vi "Select_Table_Vaule.vi"(6 "Boolean":bool, 8 "Vaule":string, 9 "Action":string, 11 "Table":string[][](array[string])) -> (0 "Result":bool, 3 "vaule":string[](array[string]))   [LabVIEW 2017]
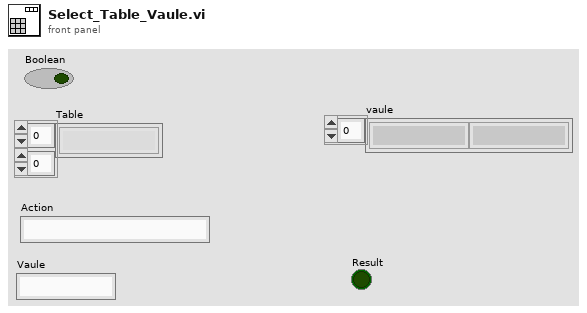
[diagram p1: front panel]
types:
  T1 = typedef "HD Config.ctl" = cluster{" PC":cluster{"PC Address":u8[], "PC Port":i32}, "FCO":cluster{"COM":refnum<visa-resource-name>, "Baudrate":u32}, "DC Power ":cluster{"COM":refnum<visa-resource-name>, "Baudrate":u32}, "PW3336":cluster{"COM":refnum<visa-resource-name>, "Baudrate":u32}, "Lefoo":cluster{"COM":refnum<visa-resource-name>, "Baudrate":u32}, "Tempt&Hum":cluster{"COM":refnum<visa-resource-name>, "Baudrate":u32}, "DIPC":cluster{"COM":refnum<visa-resource-name>}, "Daemon":cluster{"IP Address":string, "Port":u16, "Retry":u16}, "NFC_Cmd":cluster{"COM":refnum<visa-resource-name>, "Baudrate":u32}, "Fail_resume_mode":bool, "GRR":bool, "NFC _Serial":cluster{"COM":refnum<visa-resource-name>, "Baudrate":u32}}
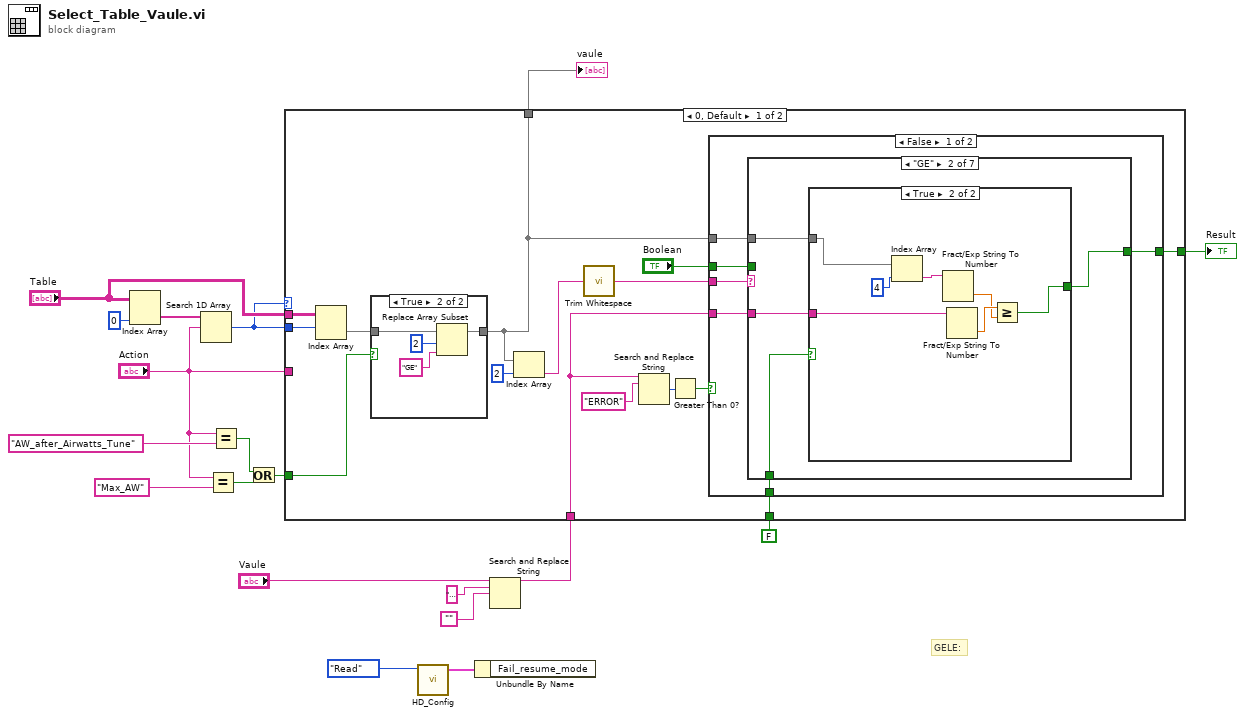
[diagram p0: block diagram]
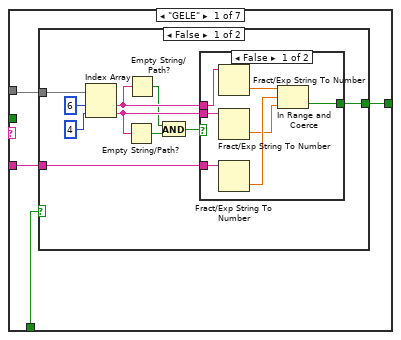
[diagram p3: hidden frame]
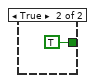
[diagram p4: hidden frame]
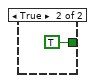
[diagram p5: hidden frame]
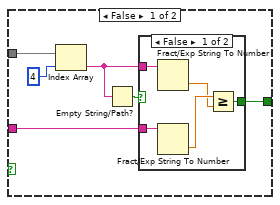
[diagram p6: hidden frame]
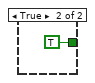
[diagram p7: hidden frame]
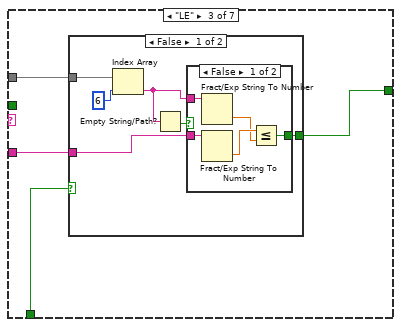
[diagram p8: hidden frame]
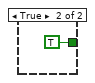
[diagram p9: hidden frame]
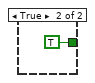
[diagram p10: hidden frame]
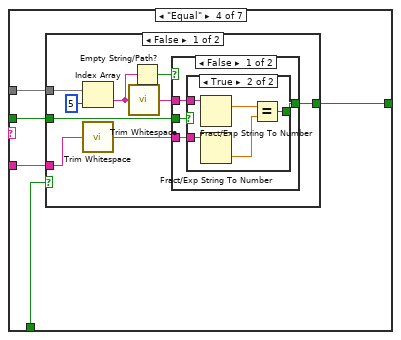
[diagram p11: hidden frame]
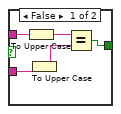
[diagram p12: hidden frame]
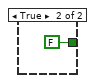
[diagram p13: hidden frame]
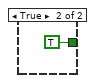
[diagram p14: hidden frame]
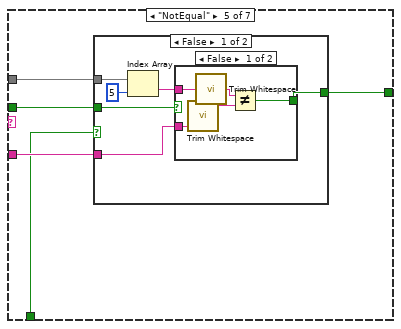
[diagram p15: hidden frame]
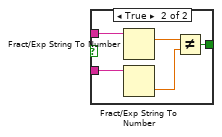
[diagram p16: hidden frame]
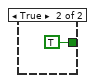
[diagram p17: hidden frame]
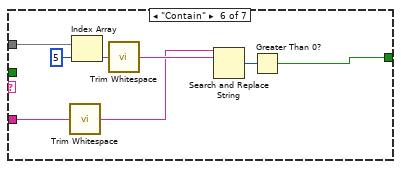
[diagram p18: hidden frame]
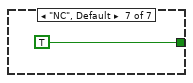
[diagram p19: hidden frame]
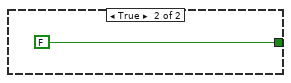
[diagram p20: hidden frame]
diagram:
  # "GELE:"
  n1 = Index Array(array="Table", index (col)=0 ("禁用的索引 (列)")) -> (element=w18:string[])  [unwired: 1 in]
  n2 = Search 1D Array(1D array=w18, element="Action") -> (index of element=w15:i32)  [unwired: 1 in]
  n3 = Equal?(x="Action", y="Max_AW") -> (x = y?=w4:bool)
  n4 = Equal?(x="Action", y="AW_after_Airwatts_Tune") -> (x = y?=w1:bool)
  n5 = Or(x=w1, y=w4) -> (x .or. y?=w3:bool)
  n6 = call "HD_Config.vi"("Step"=enum16{"Initial", "Write", "Read"}."Read") -> ("HD Config out"=w8:T1)  [unwired: 9 in, 1 out]
  n7 = Unbundle By Name(w8) -> ()  [unwired: 1 out]
  n8 = Search and Replace String(input string="Vaule", search string="\u0000", replace string="") -> (result string=w10:string)  [unwired: 5 in, 3 out]
  n9 = case shown="0, Default" w15 {
    tunnel: "Table" -> [w34 _]
    tunnel: w15 -> [w33 _]
    tunnel: w10 -> [w27 _]
    tunnel: [w29 _] -> w16
    tunnel: [w21 w172] -> w14
    tunnel: "Action" -> [_ w171]
    tunnel: FALSE ("Fail_resume_mode") -> [w23 _]
    tunnel: w3 -> [w20 _]
    frame 0, Default {
      n10 = Index Array(array=w34, index (row)=w33) -> (element=w22:string[])  [unwired: 1 in]
      n11 = case shown="True" w20 {
        tunnel: w22 -> [w35 w39]
        tunnel: [w35 w38] -> w21
        frame False {
        }
        frame True {
          n12 = Replace Array Subset ("替换数组子集")(array=w39, new element="GE" ("新元素/子数组"), index=2 ("索引")) -> (w38:string[])
        }
      }
      n13 = Index Array(array=w21, index=2 ("索引")) -> (element=w31:string)
      n14 = call <vilib>:"Trim Whitespace.vi"("string"=w31) -> ("trimmed string"=w32:string)  [unwired: 1 in]
      n15 = Search and Replace String(input string=w27, search string="ERROR") -> (number of replacements=w26:i32)  [unwired: 6 in, 3 out]
      n16 = Greater Than 0?(x=w26) -> (x > 0?=w25:bool)
      n17 = case shown="False" w25 {
        tunnel: w32 -> [w45 _]
        tunnel: [w44 FALSE] -> w29
        tunnel: w21 -> [w43 _]
        tunnel: w27 -> [w42 _]
        tunnel: "Boolean" -> [w41 _]
        tunnel: w23 -> [w40 _]
        frame False {
          n18 = case shown="\"GE\"" w45 {
            tunnel: w43 -> [w48 w71 w94 w113 w143 w167 _]
            tunnel: w42 -> [w49 w72 w95 w111 w141 w166 _]
            tunnel: [w47 w70 w93 w112 w142 w163 TRUE] -> w44
            tunnel: w41 -> [_ _ _ w110 w140 _ _]
            tunnel: w40 -> [w46 w69 w92 w109 w139 _ _]
            frame "GELE" {
              n19 = case shown="False" w46 {
                tunnel: w49 -> [w59 _]
                tunnel: w48 -> [w58 _]
                tunnel: [w55 TRUE] -> w47
                frame False {
                  n20 = Index Array(array=w58, index #1=6 ("索引"), index #2=4 ("索引")) -> (element #1=w54:string, element #2=w53:string)
                  n21 = Empty String/Path?(string/path=w53) -> (empty?=w52:bool)
                  n22 = Empty String/Path?(string/path=w54) -> (empty?=w51:bool)
                  n23 = And(x=w51, y=w52) -> (x .and. y?=w50:bool)
                  n24 = case shown="False" w50 {
                    tunnel: w59 -> [w66 _]
                    tunnel: [w62 TRUE] -> w55
                    tunnel: w54 -> [w61 _]
                    tunnel: w53 -> [w60 _]
                    frame False {
                      n25 = Fract/Exp String To Number(string=w61) -> (number=w64:dbl)  [unwired: 3 in, 1 out]
                      n26 = Fract/Exp String To Number(string=w60) -> (number=w63:dbl)  [unwired: 3 in, 1 out]
                      n27 = Fract/Exp String To Number(string=w66) -> (number=w65:dbl)  [unwired: 3 in, 1 out]
                      n28 = In Range and Coerce(upper limit=w64, x=w65, lower limit=w63) -> (In Range?=w62:bool)  [unwired: 1 out]
                    }
                    frame True {
                    }
                  }
                }
                frame True {
                }
              }
            }
            frame "GE" {
              n29 = case shown="True" w69 {
                tunnel: w72 -> [w78 w89]
                tunnel: w71 -> [w77 w90]
                tunnel: [w75 w91] -> w70
                frame False {
                  n30 = Index Array(array=w77, index=4 ("索引")) -> (element=w74:string)
                  n31 = Empty String/Path?(string/path=w74) -> (empty?=w73:bool)
                  n32 = case shown="False" w73 {
                    tunnel: w78 -> [w83 _]
                    tunnel: [w80 TRUE] -> w75
                    tunnel: w74 -> [w79 _]
                    frame False {
                      n33 = Fract/Exp String To Number(string=w79) -> (number=w81:dbl)  [unwired: 3 in, 1 out]
                      n34 = Fract/Exp String To Number(string=w83) -> (number=w82:dbl)  [unwired: 3 in, 1 out]
                      n35 = Greater Or Equal?(x=w82, y=w81) -> (x >= y?=w80:bool)
                    }
                    frame True {
                    }
                  }
                }
                frame True {
                  n36 = Index Array(array=w90, index=4 ("索引")) -> (element=w88:string)
                  n37 = Fract/Exp String To Number(string=w88) -> (number=w85:dbl)  [unwired: 3 in, 1 out]
                  n38 = Fract/Exp String To Number(string=w89) -> (number=w86:dbl)  [unwired: 3 in, 1 out]
                  n39 = Greater Or Equal?(x=w86, y=w85) -> (x >= y?=w91:bool)
                }
              }
            }
            frame "LE" {
              n40 = case shown="False" w92 {
                tunnel: w95 -> [w101 _]
                tunnel: w94 -> [w100 _]
                tunnel: [w98 TRUE] -> w93
                frame False {
                  n41 = Index Array(array=w100, index=6 ("索引")) -> (element=w97:string)
                  n42 = Empty String/Path?(string/path=w97) -> (empty?=w96:bool)
                  n43 = case shown="False" w96 {
                    tunnel: w101 -> [w106 _]
                    tunnel: [w103 TRUE] -> w98
                    tunnel: w97 -> [w102 _]
                    frame False {
                      n44 = Fract/Exp String To Number(string=w102) -> (number=w104:dbl)  [unwired: 3 in, 1 out]
                      n45 = Fract/Exp String To Number(string=w106) -> (number=w105:dbl)  [unwired: 3 in, 1 out]
                      n46 = Less Or Equal?(x=w105, y=w104) -> (x <= y?=w103:bool)
                    }
                    frame True {
                    }
                  }
                }
                frame True {
                }
              }
            }
            frame "Equal" {
              n47 = case shown="False" w109 {
                tunnel: w113 -> [w121 _]
                tunnel: [w120 TRUE] -> w112
                tunnel: w111 -> [w119 _]
                tunnel: w110 -> [w118 _]
                frame False {
                  n48 = Index Array(array=w121, index=5 ("索引")) -> (element=w117:string)
                  n49 = call <vilib>:"Trim Whitespace.vi"("string"=w119) -> ("trimmed string"=w115:string)  [unwired: 1 in]
                  n50 = call <vilib>:"Trim Whitespace.vi"("string"=w117) -> ("trimmed string"=w114:string)  [unwired: 1 in]
                  n51 = Empty String/Path?(string/path=w117) -> (empty?=w116:bool)
                  n52 = case shown="False" w116 {
                    tunnel: [w126 FALSE] -> w120
                    tunnel: w115 -> [w125 _]
                    tunnel: w118 -> [w124 _]
                    tunnel: w114 -> [w123 _]
                    frame False {
                      n53 = case shown="True" w124 {
                        tunnel: [w131 w136] -> w126
                        tunnel: w123 -> [w130 w135]
                        tunnel: w125 -> [w129 w134]
                        frame False {
                          n54 = To Upper Case(1:w130) -> (0:w128:string)
                          n55 = To Upper Case(1:w129) -> (0:w127:string)
                          n56 = Equal?(x=w128, y=w127) -> (x = y?=w131:bool)
                        }
                        frame True {
                          n57 = Fract/Exp String To Number(string=w135) -> (number=w133:dbl)  [unwired: 3 in, 1 out]
                          n58 = Fract/Exp String To Number(string=w134) -> (number=w132:dbl)  [unwired: 3 in, 1 out]
                          n59 = Equal?(x=w133, y=w132) -> (x = y?=w136:bool)
                        }
                      }
                    }
                    frame True {
                    }
                  }
                }
                frame True {
                }
              }
            }
            frame "NotEqual" {
              n60 = case shown="False" w139 {
                tunnel: w143 -> [w148 _]
                tunnel: [w147 TRUE] -> w142
                tunnel: w141 -> [w145 _]
                tunnel: w140 -> [w144 _]
                frame False {
                  n61 = Index Array(array=w148, index=5 ("索引")) -> (element=w146:string)
                  n62 = case shown="False" w144 {
                    tunnel: [w154 w159] -> w147
                    tunnel: w146 -> [w153 w158]
                    tunnel: w145 -> [w152 w157]
                    frame False {
                      n63 = call <vilib>:"Trim Whitespace.vi"("string"=w152) -> ("trimmed string"=w150:string)  [unwired: 1 in]
                      n64 = call <vilib>:"Trim Whitespace.vi"("string"=w153) -> ("trimmed string"=w151:string)  [unwired: 1 in]
                      n65 = Not Equal?(x=w151, y=w150) -> (x != y?=w154:bool)
                    }
                    frame True {
                      n66 = Fract/Exp String To Number(string=w158) -> (number=w156:dbl)  [unwired: 3 in, 1 out]
                      n67 = Fract/Exp String To Number(string=w157) -> (number=w155:dbl)  [unwired: 3 in, 1 out]
                      n68 = Not Equal?(x=w156, y=w155) -> (x != y?=w159:bool)
                    }
                  }
                }
                frame True {
                }
              }
            }
            frame "Contain" {
              n69 = call <vilib>:"Trim Whitespace.vi"("string"=w166) -> ("trimmed string"=w161:string)  [unwired: 1 in]
              n70 = Index Array(array=w167, index=5 ("索引")) -> (element=w165:string)
              n71 = call <vilib>:"Trim Whitespace.vi"("string"=w165) -> ("trimmed string"=w162:string)  [unwired: 1 in]
              n72 = Search and Replace String(input string=w161, search string=w162) -> (number of replacements=w164:i32)  [unwired: 6 in, 3 out]
              n73 = Greater Than 0?(x=w164) -> (x > 0?=w163:bool)
            }
            frame "NC", Default {
            }
          }
        }
        frame True {
        }
      }
    }
    frame -1 {
      n74 = Build Array (concatenate)(w171, string[] ["", "", "Enable", "", "", ""] ("Table")) -> (w172:string[])
    }
  }
  "Result" <- w16
  "vaule" <- w14
